vi "to string.vi"(8 "error in":errorcluster, 11 "configuration in":refnum<class "Bus Configuration.lvclass">) -> (0 "error out":errorcluster, 1 "data":string, 2 "version":string, 3 "configuration out":refnum<class "Bus Configuration.lvclass">)   [LabVIEW 2014, in "Bus Configuration.lvclass"]
doc: "Provides an interface for saving a module configuration to a file or other serialized data source. It is recommended that all children of this class store data in two sets--data required for its own initialization, and any data required for parent initialization--and that each implementation uses the <b>Call Parent Method</b> primitive to serialize parent information."
uses:
  Bus Configuration.lvclass
  Bus Configuration.lvclass/Bus Configuration.ctl
  <vilib>/NI/Configuration Framework/serializable configuration/NISE_CEF_serializable configuration.lvclass
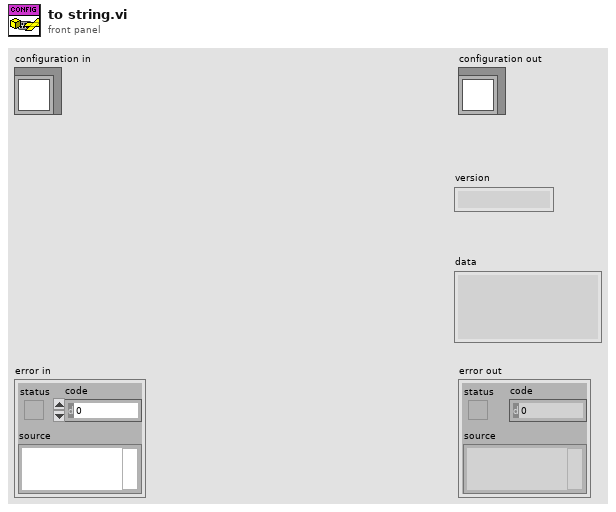
[diagram p1: front panel]
types:
  T1 = typedef "Bus Configuration.lvclass/SPI Configuration.ctl" = cluster{"SCLK":string, "MOSI":string, "MISO":string}
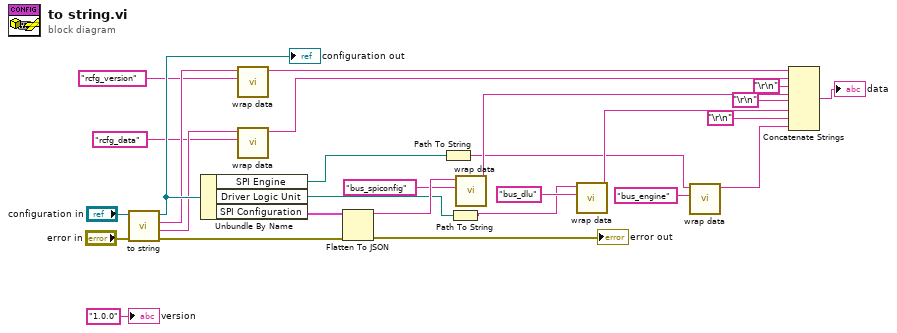
[diagram p0: block diagram]
diagram:
  n1 = call-parent "to string.vi"("error in"="error in", "configuration in"="configuration in") -> ("error out"=w24:errorcluster, "data"=w20:string, "version"=w21:string, "configuration out"=w26:refnum<class "Bus Configuration.lvclass">)  [unwired: 6 in]
  "configuration out" <- w26
  n2 = Unbundle By Name(w26) -> ("SPI Engine"=w2:path, "Driver Logic Unit"=w8:path, "SPI Configuration"=w25:T1)
  n3 = call <vilib>:"wrap data.vi"("identifier"="rcfg_version", "data to wrap"=w21) -> ("wrapped data"=w16:string)  [unwired: 9 in]
  n4 = call <vilib>:"wrap data.vi"("identifier"="rcfg_data", "data to wrap"=w20) -> ("wrapped data"=w15:string)  [unwired: 9 in]
  n5 = Flatten To JSON(anything=w25, error in (no error)=w24) -> (JSON string=w23:string, 11:→"error out":errorcluster)  [unwired: 1 in]
  n6 = Path To String(path=w2) -> (string=w1:string)
  n7 = Path To String(path=w8) -> (string=w7:string)
  n8 = call <vilib>:"wrap data.vi"("identifier"="bus_spiconfig", "data to wrap"=w23) -> ("wrapped data"=w13:string)  [unwired: 9 in]
  n9 = call <vilib>:"wrap data.vi"("identifier"="bus_dlu", "data to wrap"=w7) -> ("wrapped data"=w9:string)  [unwired: 9 in]
  n10 = call <vilib>:"wrap data.vi"("identifier"="bus_engine", "data to wrap"=w1) -> ("wrapped data"=w3:string)  [unwired: 9 in]
  n11 = Concatenate Strings(w16, w15, "\r\n", w13, "\r\n", w9, "\r\n", w3) -> (→"data":string)
  "version" <- "1.0.0" ("version")
